vi "set Max Lines Per Log File.vi"(11 "Max Lines Per Log File":i32) -> ()   [LabVIEW 2015, in "System Config.lvclass"]
uses:
  System Config.lvclass
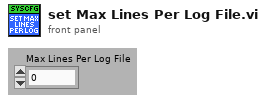
[diagram p1: front panel]
types:
  T1 = typedef "System Config.lvclass/ClassAttributesRef.ctl" = refnum<data-value>
  T2 = typedef "System Config.lvclass/ClassAttributes.ctl" = cluster{"Config":cluster{"Logging":cluster{"Log Files Directory":path, "Max Lines Per Log File":i32}, "Settings":T3}, "Core":cluster{"Config Directory":path, "Name":string, "Config Changed":refnum<user-event>}}
  T3 = typedef "System Config.lvclass/Settings.ctl" = cluster{"Dummy":dbl}
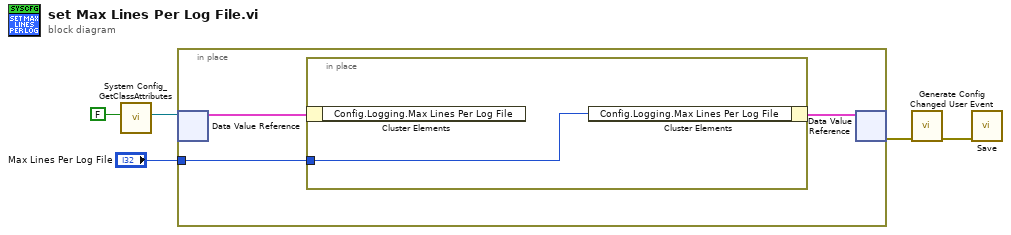
[diagram p0: block diagram]
diagram:
  n1 = call "System Config_GetClassAttributes.vi"("return data? (T)"=FALSE ("return data")) -> ("class attributes ref"=w4:T1)  [unwired: 7 in, 3 out]
  n2 = in-place {
    in-place-border: "Max Lines Per Log File" -> [w6]
    n3 = in-place-dvr #1(w4) -> (w7:T2)  [unwired: 1 out]
    n4 = in-place {
      in-place-border: w6 -> [w9]
      n5 = in-place-cluster #2(w7) -> ()  [unwired: 1 out]
      n6 = in-place-cluster #2("Config.Logging.Max Lines Per Log File"=w9) -> (w8:T2)
    }
    n7 = in-place-dvr #1(w8) -> (w2:errorcluster)  [unwired: 1 out]
  }
  n8 = call "Generate Config Changed User Event.vi"("error in (no error)"=w2) -> ("error out"=w1:errorcluster)  [unwired: 10 in]
  n9 = call "Save.vi"("error in (no error)"=w1) -> ()  [unwired: 10 in, 1 out]
